vi "Test CQuant DLL.vi"() -> ()   [LabVIEW 2015]
uses:
  C:/Distributed/CalFlex.dll
  CalFlex.dll
panel:
  out "yR":dbl
  out "r2":dbl
  out "coefficients":dbl[](array[numeric])
  out "error out":errorcluster
  out "isValid":bool
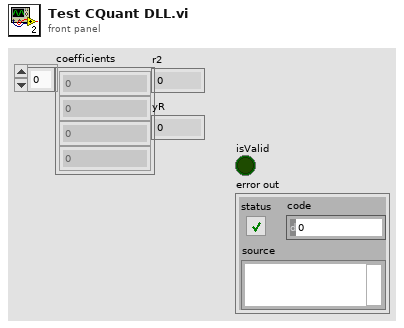
[diagram p1: front panel]
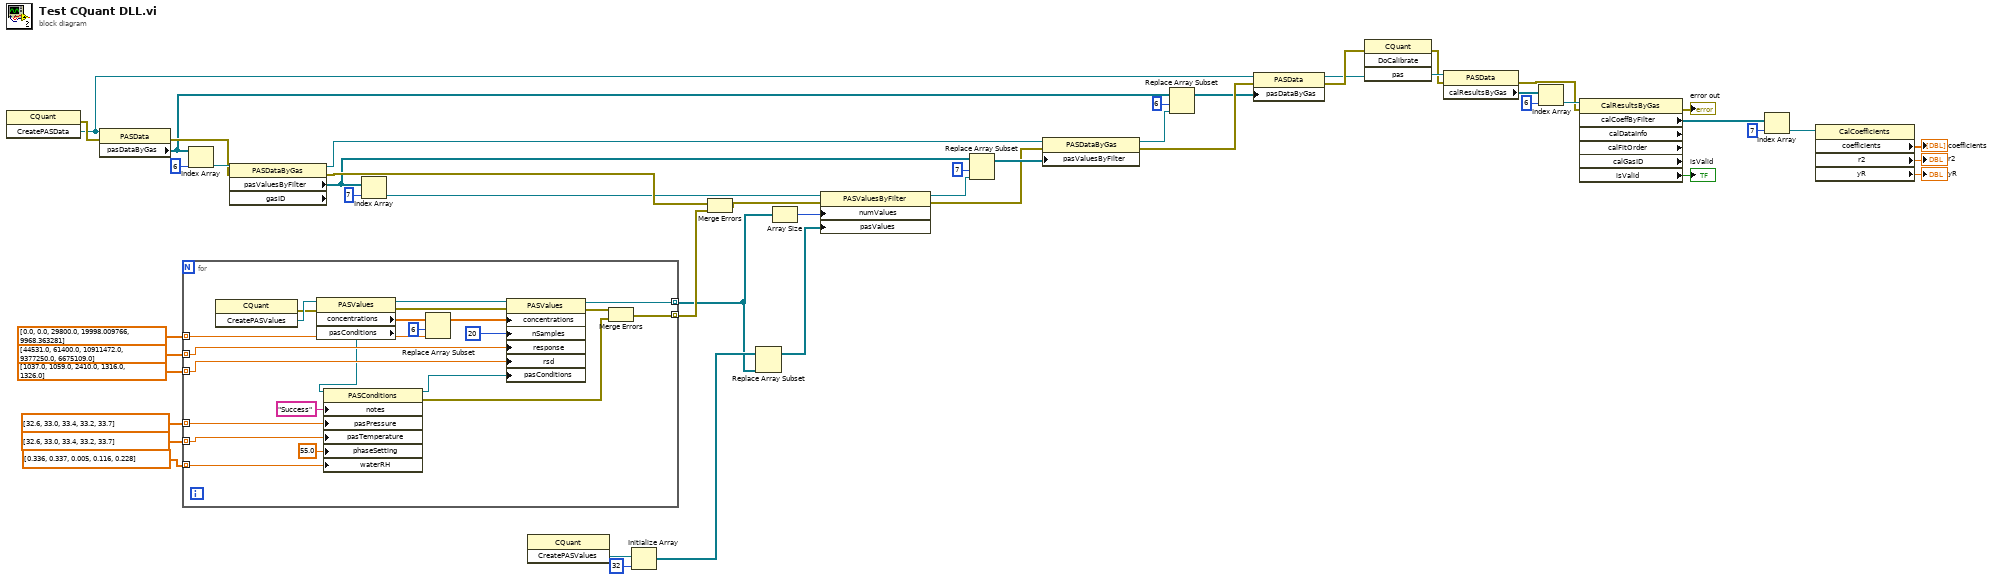
[diagram p0: block diagram]
diagram:
  n1 = invoke class="CQuant" method="CreatePASData"() -> (error out=w49:errorcluster, "CreatePASData"=w14:refnum<k24>)  [unwired: 3 in, 1 out]
  n2 = property class="PASData"(reference=w14, error in=w49) -> (error out=w39:errorcluster, "pasDataByGas"=w28:refnum<k24>[])  [unwired: 1 out]
  n3 = for {
    tunnel: dbl[] [0.0, 0.0, 29800.0, 19998.009766, 9968.363281] ("concentrations") -> [w69] mode=indexing
    tunnel: dbl[] [44531.0, 61400.0, 10911472.0, 9377250.0, 6675109.0] ("concentrations") -> [w63] mode=indexing
    tunnel: dbl[] [1037.0, 1059.0, 2410.0, 1316.0, 1326.0] ("concentrations") -> [w62] mode=indexing
    tunnel: dbl[] [32.6, 33.0, 33.4, 33.2, 33.7] ("concentrations") -> [w61] mode=indexing
    tunnel: dbl[] [32.6, 33.0, 33.4, 33.2, 33.7] ("concentrations") -> [w60] mode=indexing
    tunnel: dbl[] [0.336, 0.337, 0.005, 0.116, 0.228] ("concentrations") -> [w58] mode=indexing
    tunnel: [w66] -> w8 mode=indexing
    tunnel: [w53] -> w38 mode=indexing
    n4 = invoke class="CQuant" method="CreatePASValues"() -> (error out=w50:errorcluster, "CreatePASValues"=w51:refnum<k24>)  [unwired: 3 in, 1 out]
    n5 = property class="PASValues"(reference=w51, error in=w50) -> (reference out=w68:refnum<k24>, error out=w67:errorcluster, "concentrations"=w71:dbl[], "pasConditions"=w52:refnum<k24>)
    n6 = property class="PASConditions"(reference=w52, "notes"="Success", "pasPressure"=w61, "pasTemperature"=w60, "phaseSetting"=55.0, "waterRH"=w58) -> (reference out=w55:refnum<k24>, error out=w56:errorcluster)  [unwired: 1 in]
    n7 = Replace Array Subset(array=w71, new element=w69, index=6) -> (w65:dbl[])
    n8 = property class="PASValues"(reference=w68, error in=w67, "concentrations"=w65, "nSamples"=20, "response"=w63, "rsd"=w62, "pasConditions"=w55) -> (reference out=w66:refnum<k24>, error out=w57:errorcluster)
    n9 = Merge Errors(w57, w56) -> (w53:errorcluster)
  }
  n10 = Index Array(array=w28, index=6) -> (element=w47:refnum<k24>)
  n11 = property class="PASDataByGas" props=["pasValuesByFilter", "gasID"](reference=w47, error in=w39) -> (reference out=w32:refnum<k24>, error out=w36:errorcluster, "pasValuesByFilter"=w34:refnum<k24>[])  [unwired: 1 out]
  n12 = Index Array(array=w34, index=7) -> (element=w35:refnum<k24>)
  n13 = invoke class="CQuant" method="CreatePASValues"() -> ("CreatePASValues"=w11:refnum<k24>)  [unwired: 3 in, 2 out]
  n14 = Initialize Array(w11, 32 ("dimension size")) -> (w9:refnum<k24>[])
  n15 = Merge Errors(w36, w38) -> (w37:errorcluster)
  n16 = Replace Array Subset(array=w9, new element=w8) -> (w7:refnum<k24>[])  [unwired: 1 in]
  n17 = Array Size(array=w8) -> (size(s)=w12:i32)
  n18 = property class="PASValuesByFilter"(reference=w35, error in=w37, "numValues"=w12, "pasValues"=w7) -> (reference out=w15:refnum<k24>, error out=w30:errorcluster)
  n19 = Replace Array Subset(array=w34, new element=w15, index=7) -> (w31:refnum<k24>[])
  n20 = property class="PASDataByGas"(reference=w32, error in=w30, "pasValuesByFilter"=w31) -> (reference out=w27:refnum<k24>, error out=w26:errorcluster)
  n21 = Replace Array Subset(array=w28, new element=w27, index=6) -> (w25:refnum<k24>[])
  n22 = property class="PASData"(reference=w14, error in=w26, "pasDataByGas"=w25) -> (reference out=w13:refnum<k24>, error out=w24:errorcluster)
  n23 = invoke class="CQuant" method="DoCalibrate"(error in=w24, "pas"=w13) -> (error out=w18:errorcluster, "pas"=w23:refnum<k24>)  [unwired: 2 in, 2 out]
  n24 = property class="PASData"(reference=w23, error in=w18) -> (error out=w17:errorcluster, "calResultsByGas"=w22:refnum<k24>[])  [unwired: 1 out]
  n25 = Index Array(array=w22, index=6) -> (element=w20:refnum<k24>)
  n26 = property class="CalResultsByGas" props=["calCoeffByFilter", "calDataInfo", "calFitOrder", "calGasID", "isValid"](reference=w20, error in=w17) -> (error out=→"error out":errorcluster, "calCoeffByFilter"=w6:refnum<k24>[], "isValid"=→"isValid":bool)  [unwired: 4 out]
  n27 = Index Array(array=w6, index=7) -> (element=w4:refnum<k24>)
  n28 = property class="CalCoefficients"(reference=w4) -> ("coefficients"=→"coefficients":dbl[], "r2"=→"r2":dbl, "yR"=→"yR":dbl)  [unwired: 1 in, 2 out]
